vi "Remove Pref Hierarchy.vi"(8 "error in (no error)":errorcluster, 10 "Pref Hierarchy":string[](array[string]), 11 "Pref Group in":refnum<class "Pref Group.lvclass">) -> (0 "error out":errorcluster, 3 "Pref Group out":refnum<class "Pref Group.lvclass">)   [LabVIEW 2020, in "User Prefs.lvlib" / "Pref Group.lvclass"]
uses:
  Pref Group.lvclass
  Pref Group.lvclass/Pref Group.ctl
  lv-cdm/CDM-Config/Config Manager/Config Manager.lvclass
  lv-cdm/CDM-Config/Config Element/Config Element.lvclass
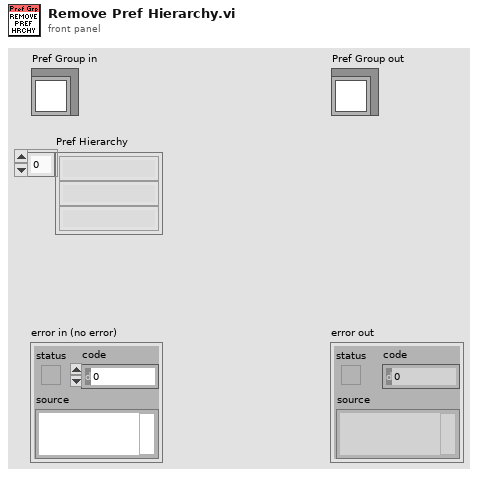
[diagram p1: front panel]
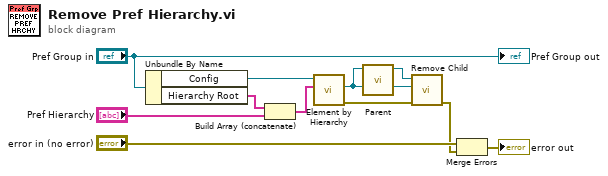
[diagram p0: block diagram]
diagram:
  n1 = Unbundle By Name("Pref Group in") -> ("Config"=w7:refnum<class "Config Manager.lvclass">, "Hierarchy Root"=w9:string[])
  n2 = Build Array (concatenate)(w9, "Pref Hierarchy") -> (w6:string[])
  n3 = call "Element by Hierarchy.vi"("Hierarchy"=w6, "Config Manager in"=w7) -> ("error out"=w3:errorcluster, "Config Element"=w4:refnum<class "Config Element.lvclass">)  [unwired: 7 in, 1 out]
  n4 = call "Parent.vi"("Config Element in"=w4) -> ("Parent"=w5:refnum<class "Config Element.lvclass">)  [unwired: 9 in, 1 out]
  n5 = call "Remove Child.vi"("error in (no error)"=w3, "Child"=w4, "Config Element in"=w5) -> ("error out"=w1:errorcluster)  [unwired: 7 in, 1 out]
  n6 = Merge Errors("error in (no error)", w1) -> (→"error out":errorcluster)
  "Pref Group out" <- "Pref Group in"
